vi "GetEXT.vi"(5 "format string (%_20f)":string="%_20f", 7 "key description":string, 8 "sections":string[](array[string]), 9 "numeric":ext, 11 "info data":string) -> (0 "sections out":string[](array[string]), 2 "value":ext format="%#_20g", 3 "info data out":string)   [LabVIEW 2019, in "infolib.lvlib"]
doc: "Add a new numeric key to Info Data string. If section exists in Info Data string, inserts key into this section."
uses:
  infolib.lvlib
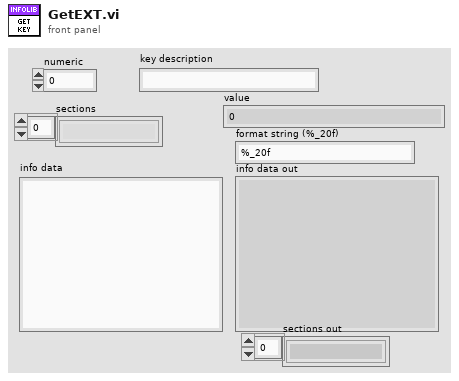
[diagram p1: front panel]
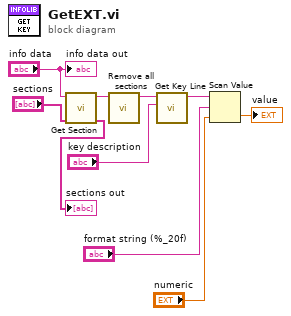
[diagram p0: block diagram]
diagram:
  n1 = call "Get Section.vi"("sections"="sections", "info data"="info data") -> ("sections out"=→"sections out":string[], "section part"=w10:string)  [unwired: 7 in, 1 out]
  n2 = call "Remove all sections.vi"("info data"=w10) -> ("info data out"=w9:string)  [unwired: 10 in]
  n3 = call "Get Key Line.vi"("key description"="key description", "info data"=w9) -> ("key value"=w5:string)  [unwired: 9 in]
  n4 = Scan Value(string=w5, format string="format string (%_20f)", default (0 dbl)="numeric") -> (value=→"value":ext)  [unwired: 1 out]
  "info data out" <- "info data"
